vi "G#BaseClass1_Create.vi"(0 "reference in":refnum<class "G#BaseClass1.lvclass">, 1 "object name":string, 4 "no registration":bool, 5 "error in (no error)":errorcluster, 6 "create method":T1=enum."Create or look up existing", 7 "user counter":bool=TRUE) -> (12 "created new?":bool, 14 "reference out":refnum<class "G#BaseClass1.lvclass">, 19 "error out":errorcluster)   [LabVIEW 2010, in "G#BaseClass1.lvclass"]
doc: "Constructor."
uses:
  G#BaseClass1.lvclass
  <vilib>/addons/_AddQ/G#Object/utils/G#Object_CreateMethod.ctl
  <vilib>/addons/_AddQ/G#Object/G#Object.lvclass
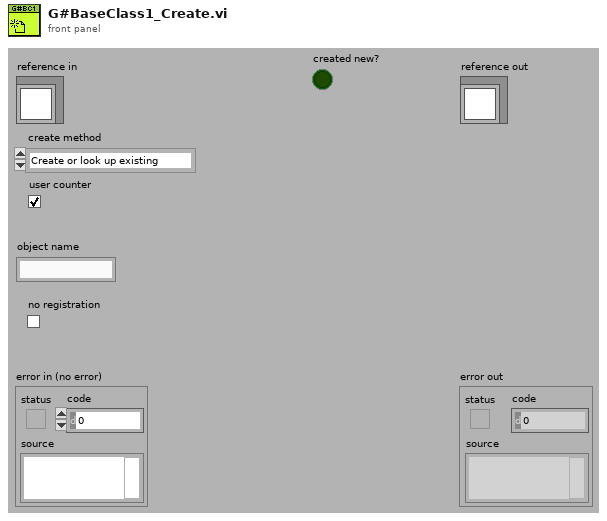
[diagram p1: front panel]
types:
  T1 = typedef "G#Object.lvclass/G#Object_CreateMethod.ctl" = enum16{"Create", "Create or look up existing", "Look up existing"}
  T2 = typedef "G#BaseClass1.lvclass/ObjectAttributesRef.ctl" = refnum<data-value>
  T3 = typedef "G#BaseClass1.lvclass/ObjectAttributes.ctl" = cluster{"Numeric":dbl, "Array":dbl[]}
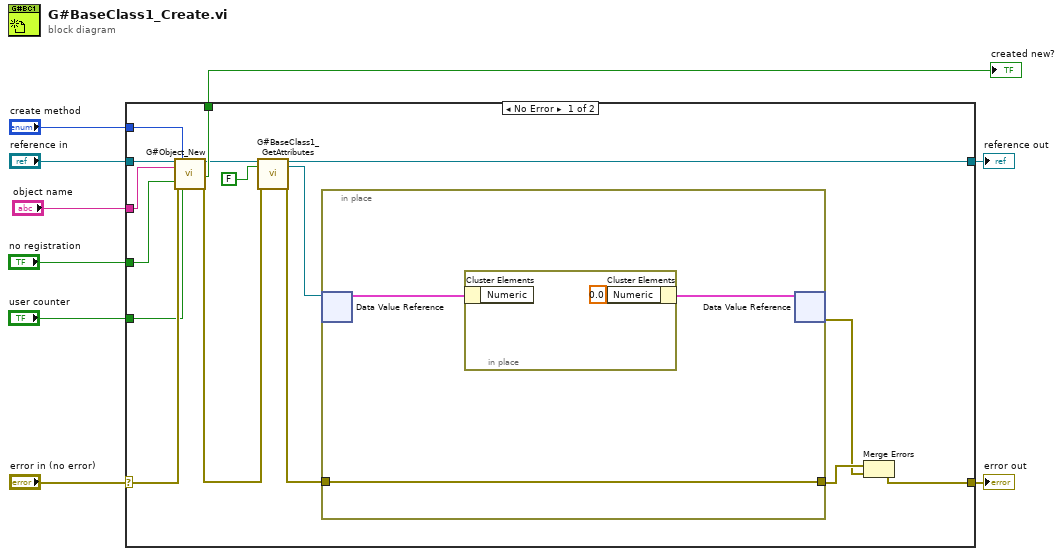
[diagram p0: block diagram]
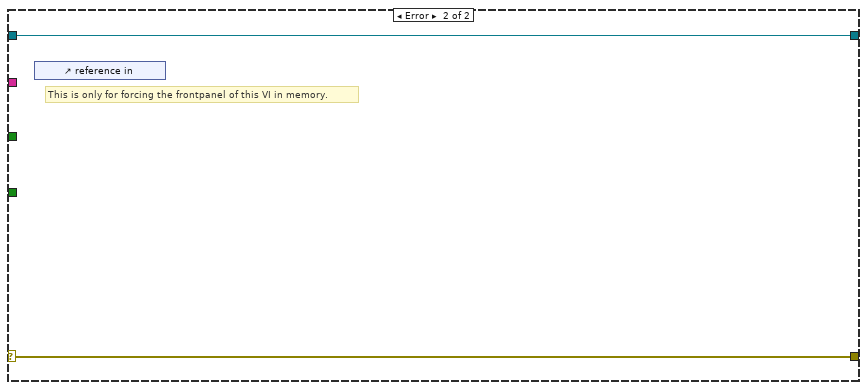
[diagram p2: hidden frame]
diagram:
  n1 = case shown="No Error" "error in (no error)" {
    selector: "error in (no error)" -> [w24 w31]
    tunnel: [w17 w31] -> w8
    tunnel: [w14 w30] -> w6
    tunnel: "reference in" -> [w25 w30]
    tunnel: "create method" -> [w21 _]
    tunnel: "object name" -> [w20 _]
    tunnel: "no registration" -> [w19 _]
    tunnel: "user counter" -> [w18 _]
    tunnel: [w16 _] -> w1
    frame No Error {
      n2 = call <vilib>:"G#Object_New.vi"("reference in"=w25, "object name"=w20, "no registration? (F)"=w19, "error in (no error)"=w24, "create method"=w21, "user counter (T)?"=w18) -> ("reference out"=w15:refnum<class "G#BaseClass1.lvclass">, "created new?"=w16:bool, "error out"=w13:errorcluster)  [unwired: 11 in]
      n3 = call "G#BaseClass1_GetAttributes.vi"("reference in"=w15, "return data? (T)"=FALSE, "error in (no error)"=w13) -> ("reference out"=w14:refnum<class "G#BaseClass1.lvclass">, "attributes ref"=w11:T2, "error out"=w12:errorcluster)  [unwired: 13 in, 1 out]
      n4 = in-place {
        in-place-border: w12 -> [w26]
        in-place-border: [w26] -> w23
        n5 = in-place-dvr #1(w11) -> (w27:T3)  [unwired: 1 out]
        n6 = in-place {
          n7 = in-place-cluster #2(w27) -> ()  [unwired: 1 out]
          n8 = in-place-cluster #2("Numeric"=0.0) -> (w28:T3)
        }
        n9 = in-place-dvr #1(w28) -> (w22:errorcluster)  [unwired: 1 out]
      }
      n10 = Merge Errors(w23, w22) -> (w17:errorcluster)
    }
    frame Error {
      # "This is only for forcing the frontpanel of this VI in memory."
      n11 = control-ref of="reference in"() -> ()  [unwired: 1 out]
    }
  }
  "error out" <- w8
  "reference out" <- w6
  "created new?" <- w1
